vi "Test GL Attributes.vi"() -> ()   [LabVIEW 2012]
uses:
  DLL/SDL.dll
  mySDL.lvlib
panel:
  out "Error":string
  out "return type 2":i32
  out "return type":i32
  out "value":i32
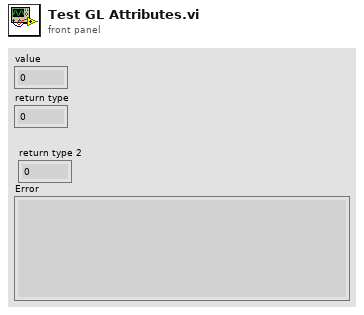
[diagram p1: front panel]
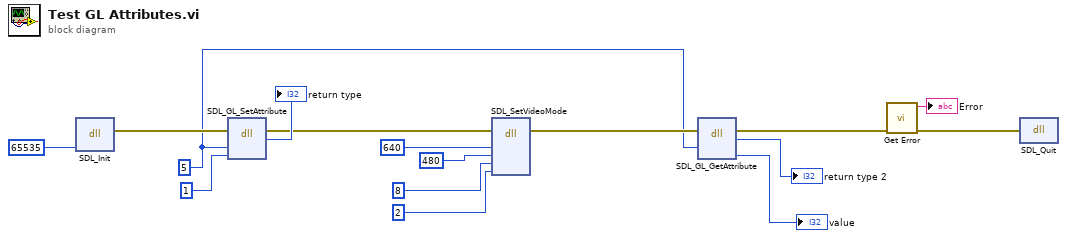
[diagram p0: block diagram]
diagram:
  w1 = u32 5 ("attribute")
  n1 = dll-call lib="C:/dev/SDL/LabVIEW/DLL/SDL.dll" fn="SDL_Init"("flags"=u32 65535 ("Flags")) -> (error out=w15:errorcluster)  [unwired: 5 in, 1 out]
  n2 = dll-call lib="C:/dev/SDL/LabVIEW/DLL/SDL.dll" fn="SDL_GL_SetAttribute"(error in=w15, "attribute"=w1, "value"=1) -> (error out=w3:errorcluster, "return type"=→"return type":i32)  [unwired: 4 in, 1 out]
  n3 = dll-call lib="C:/dev/SDL/LabVIEW/DLL/SDL.dll" fn="SDL_SetVideoMode"(error in=w3, "width"=640 ("Width"), "height"=480 ("Height"), "bpp"=8 ("BPP"), "flags"=u32 2 ("Flags")) -> (error out=w2:errorcluster)  [unwired: 7 in, 1 out]
  n4 = dll-call lib="C:/dev/SDL/LabVIEW/DLL/SDL.dll" fn="SDL_GL_GetAttribute"(error in=w2, "attribute"=w1) -> (error out=w8:errorcluster, "return type"=→"return type 2":i32, "value"=→"value":i32)  [unwired: 4 in, 1 out]
  n5 = call "Get Error.vi"("error in"=w8) -> ("error out"=w10:errorcluster, "Error"=→"Error":string)  [unwired: 9 in]
  n6 = dll-call lib="C:/dev/SDL/LabVIEW/DLL/SDL.dll" fn="SDL_Quit"(error in=w10) -> ()  [unwired: 3 in, 2 out]
